vi "Ex_WiringPi_Blinking LED.vi"(8 "error in (no error)":errorcluster) -> (0 "error out":errorcluster)   [LabVIEW 2014]
uses:
  vi.lib/Q-WaveSystems/QwaveSys Raspberry Pi for LabVIEW Home-Education/WiringPi/WiringPi Pin Mode.ctl
  vi.lib/Q-WaveSystems/QwaveSys Raspberry Pi for LabVIEW Home-Education/WiringPi/WiringPi GPIO TypeDef.ctl
  vi.lib/Q-WaveSystems/QwaveSys Raspberry Pi for LabVIEW Home-Education/QwaveSys Raspberry Pi Library.lvlib
panel:
  in  "WiringPi GPIO":T1=7 items=["SDA(I2C)-3"=8, "SCL(I2C)-5"=9, "MOSI(SPI)-19"=12, "MISO(SPI)-21"=13, "SCLK(SPI)-23"=14, "GPIO2-13"=2, "GPIO3-15"=3, "GPIO4-16"=4, "GPIO5-18"=5, "GPIO6-22"=6, "GPIO7-7"=7, "GPIO21-29"=21, "GPIO22-31"=22, "GPIO25-37"=25, "GPIO27-36"=27, "GPIO26(PWM0)-32"=26, "GPIO1(PWM0-12)"=1, "GPIO23(PWM1)-14"=23, "GPIO24(PWM1)-35"=24, "TXD(UART)-8"=15, "RXD(UART)-10"=16, "GPIO10(CE0-SPI)-24"=10, "GPPI11(CE1)-SPI)-26"=11, "GPIO28(PCM_DIN)36"=28, "GPIO29(PCM_DOUT)40"=29]
  in  "Pin Mode":T2=enum."OUTPUT"
  out "LED":bool
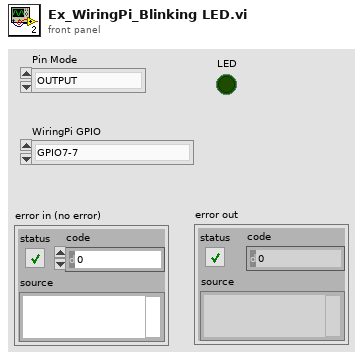
[diagram p1: front panel]
types:
  T1 = typedef "QwaveSys Raspberry Pi Library.lvlib/WiringPi GPIO TypeDef.ctl" = u8
  T2 = typedef "QwaveSys Raspberry Pi Library.lvlib/WiringPi Pin Mode.ctl" = enum8{"INPUT", "OUTPUT", "PWM_OUTPUT", "GPIO_CLOCK", "SOFT_PWM_OUTPUT", "SOFT_TONE_OUTPUT", "PWM_TONE_OUTPUT"}
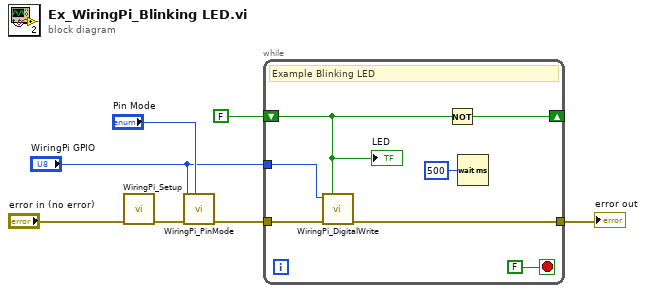
[diagram p0: block diagram]
diagram:
  n1 = call "WiringPi_Setup.vi"("error in (no error)"="error in (no error)") -> ("error out"=w6:errorcluster)  [unwired: 10 in]
  n2 = call "WiringPi_PinMode.vi"("Pin Mode"="Pin Mode", "error in (no error)"=w6, "WiringPi GPIO"="WiringPi GPIO") -> ("error out"=w5:errorcluster)  [unwired: 8 in]
  n3 = while {
    tunnel: w5 -> [w14]
    tunnel: [w12] -> w2
    shift-right: [w11] -> _
    shift-left: FALSE -> [w10]
    tunnel: "WiringPi GPIO" -> [w8]
    stop <- FALSE stop-if-true
    # "Example Blinking LED"
    n4 = call "WiringPi_DigitalWrite.vi"("Value"=w10, "error in (no error)"=w14, "WiringPi GPIO"=w8) -> ("error out"=w12:errorcluster)  [unwired: 8 in]
    n5 = Not(x=w10) -> (.not. x?=w11:bool)
    n6 = Wait (ms)(milliseconds to wait=u32 500) -> ()  [unwired: 1 out]
    "LED" <- w10
  }
  "error out" <- w2
